vi "arreglos.vi"() -> ()   [LabVIEW 2020]
panel:
  out "Array 2":string[](array[string])
  out "Motore Descortezador":dbl[](array[slide]) scale=0.0..100.0
  in  "Array":dbl[](array[slide]) scale=0.0..100.0
  # "Linea Marco"
  # "Linea area"
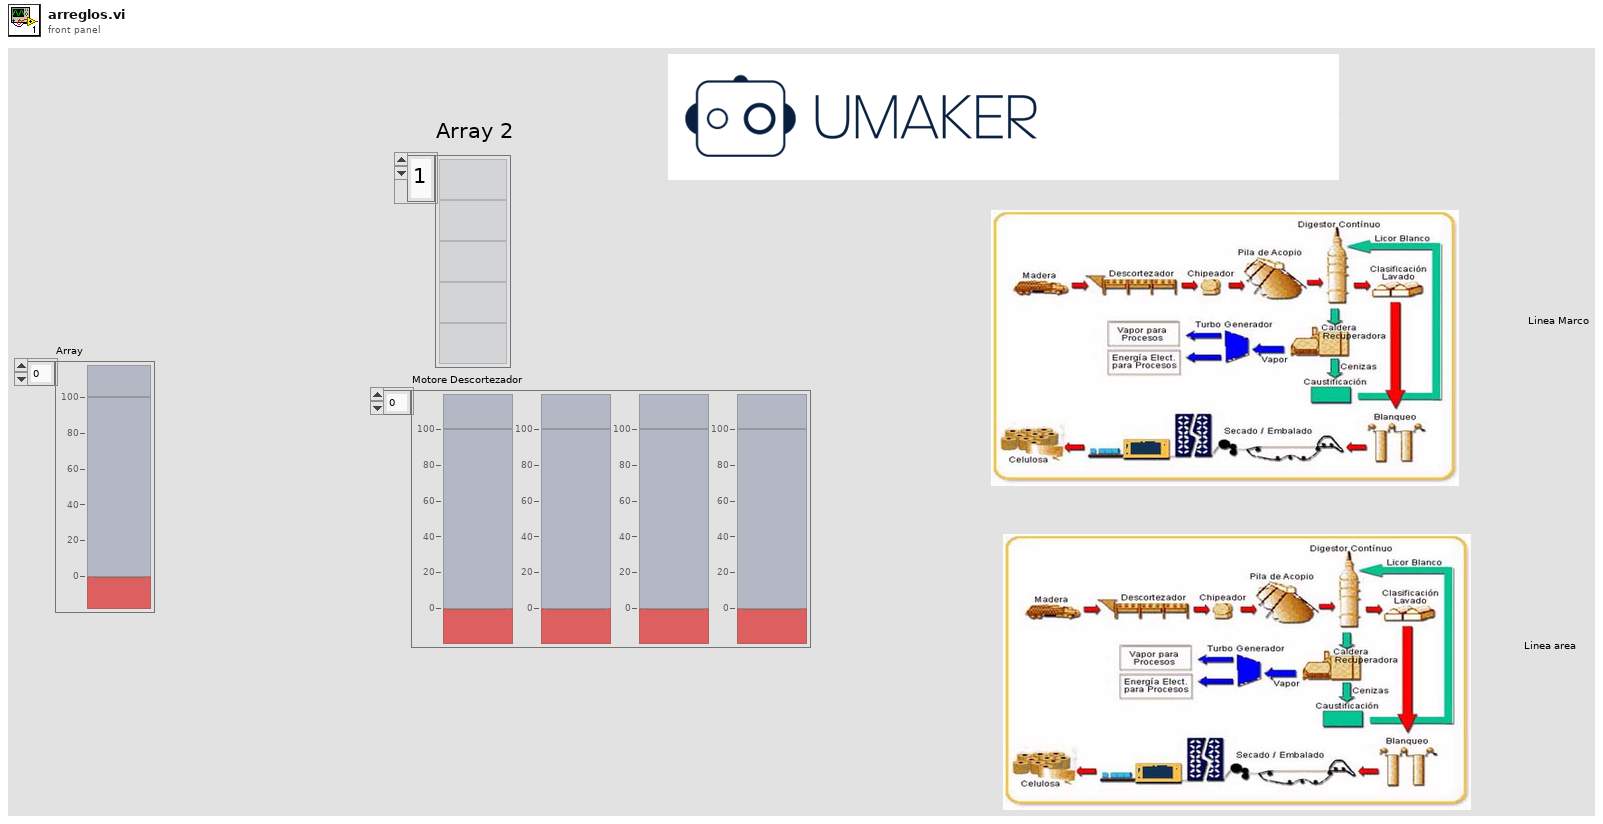
[diagram p1: front panel]
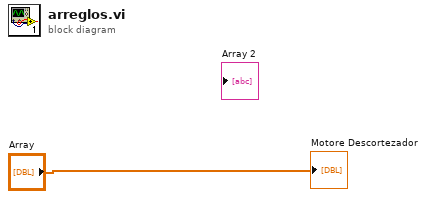
[diagram p0: block diagram]
diagram:
  "Motore Descortezador" <- "Array"
